vi "MainWashingMachine.vi"() -> ()   [LabVIEW 2020]
uses:
  Typedefinitons/type_cluster_WashingMachineDrum.ctl
panel:
  in  "Power":bool
  in  "Wallet":T1
  in  "Start Program 2":bool
  out "Process":u8(slide) scale=0.0..100.0
  out "Budget":dbl
  in  "Start Program":bool
  out "Speed rpm":dbl=20.0 min=20.0 max=60.0 step=10.0
  in  "ProgramSelection":T2(radio)
  out "status":string
  out "Temperature C°":dbl=20.0 min=20.0 max=60.0 step=10.0
  out "Cluster":T3
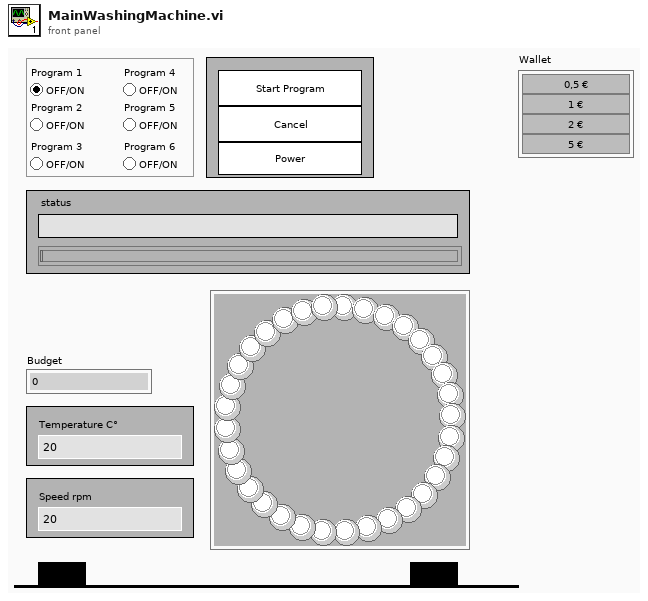
[diagram p1: front panel]
types:
  T1 = cluster{"0,50_Euro":bool, "1_Euro":bool, "2_Euro":bool, "5_Euro":bool}
  T2 = enum32{"Program 1", "Program 2", "Program 3", "Program 4", "Program 5", "Program 6"}
  T3 = typedef "type_cluster_WashingMachineDrum.ctl" = cluster{"Boolean":bool, "Boolean 2":bool, "Boolean 3":bool, "Boolean 4":bool, "Boolean 5":bool, "Boolean 6":bool, "Boolean 7":bool, "Boolean 8":bool, "Boolean 9":bool, "Boolean 10":bool, "Boolean 11":bool, "Boolean 12":bool, "Boolean 13":bool, "Boolean 14":bool, "Boolean 15":bool, "Boolean 16":bool, "Boolean 17":bool, "Boolean 18":bool, "Boolean 19":bool, "Boolean 20":bool, "Boolean 21":bool, "Boolean 22":bool, "Boolean 23":bool, "Boolean 24":bool, "Boolean 25":bool, "Boolean 26":bool, "Boolean 27":bool, "Boolean 28":bool, "Boolean 29":bool, "Boolean 30":bool, "Boolean 31":bool, "Boolean 32":bool, "Boolean 33":bool}
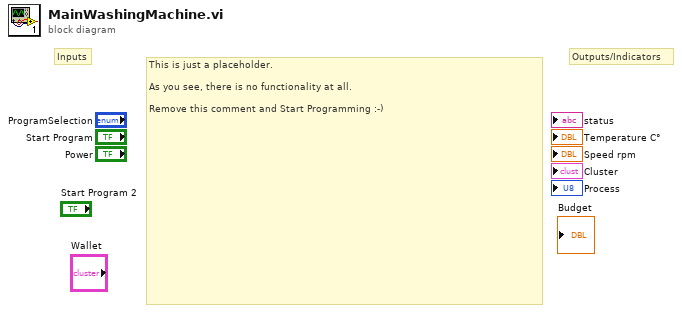
[diagram p0: block diagram]
diagram:
  # "Outputs/Indicators"
  # "Inputs"
  # "This is just a placeholder.\n\nAs you see, there is no functionality at all. \n\nRemove this comment and Start Programming :-)"
